vi "Accumulated Angle.vi"(11 "Angle In":dbl) -> (3 "Fixed Angle":dbl)   [LabVIEW 2016]
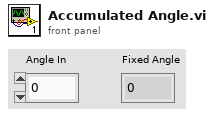
[diagram p1: front panel]
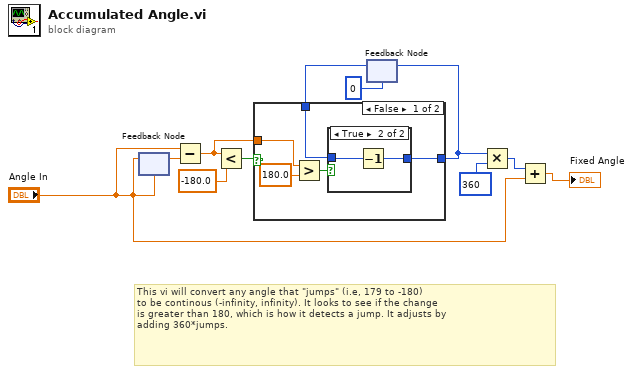
[diagram p0: block diagram]
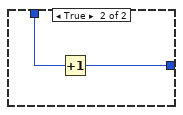
[diagram p3: hidden frame]
diagram:
  # "This vi will convert any angle that \"jumps\" (i.e, 179 to -180)\nto be continous (-infinity, infinity). It looks to see if the change\nis greater than 180, which is how it detects a jump. It adjusts by\nadding 360*jumps."
  n1 = feedback #1("Angle In") -> (w11:dbl)
  n2 = feedback-in #1("Angle In") -> ()
  n3 = Subtract(x="Angle In", y=w11) -> (x-y=w6:dbl)
  n4 = Less?(x=w6, y=-180.0) -> (x < y?=w9:bool)
  n5 = feedback #2(0) -> (w7:i32)
  n6 = case shown="False" w9 {
    tunnel: [w12 w21] -> w5
    tunnel: w7 -> [w13 w20]
    tunnel: w6 -> [w16 _]
    frame False {
      n7 = Greater?(x=w16, y=180.0) -> (0:w14:bool)
      n8 = case shown="True" w14 {
        tunnel: w13 -> [w17 w19]
        tunnel: [w17 w18] -> w12
        frame False {
        }
        frame True {
          n9 = Decrement(x=w19) -> (x-1=w18:i32)
        }
      }
    }
    frame True {
      n10 = Increment(x=w20) -> (x+1=w21:i32)
    }
  }
  n11 = feedback-in #2(w5) -> ()
  n12 = Multiply(x=w5, y=360) -> (x*y=w3:i32)
  n13 = Add(x=w3, y="Angle In") -> (x+y=→"Fixed Angle":dbl)
